vi "LDA_Analysis.vi"() -> (5 "Plug in titles":string[](array[string]), 7 "Plug in values":string[](array[string]))   [LabVIEW 2011]
uses:
  Controls/Save_Data.ctl
  Globals/LDA_meas_global_1.vi
  Globals/Plug_in_data_global.vi
  Globals/Meas_global.vi
  Globals/Constants_global.vi
  <vilib>/Analysis/NI_AALBase.lvlib
panel:
  in  "File Extension":string=".xls"
  out "Delta f":dbl
  in  "Refined Spectra":bool
  in  "No of estimates output":i32=300
  out "Autocorrelation":cluster{dbl, dbl, dbl[]}[](graph)
  in  "Mode":enum16{"Spectra", "Autocorrelation"}(ring)
  in  "Separation Character":string="\t"
  in  "Precision":i16=2
  out "Ch names":string[](array[string])
  out "Number or Good blocks":i32
  out "Resampled block length":i32
  out "Resampling Frequency":dbl
  in  "Output Directory":path
  in  "File":T1=enum."Save Data"
  out "Frequency Spectrum":cluster{dbl, dbl, dbl[]}[](graph)
  # "You must have just these two indicators on the connector pane of the vi"
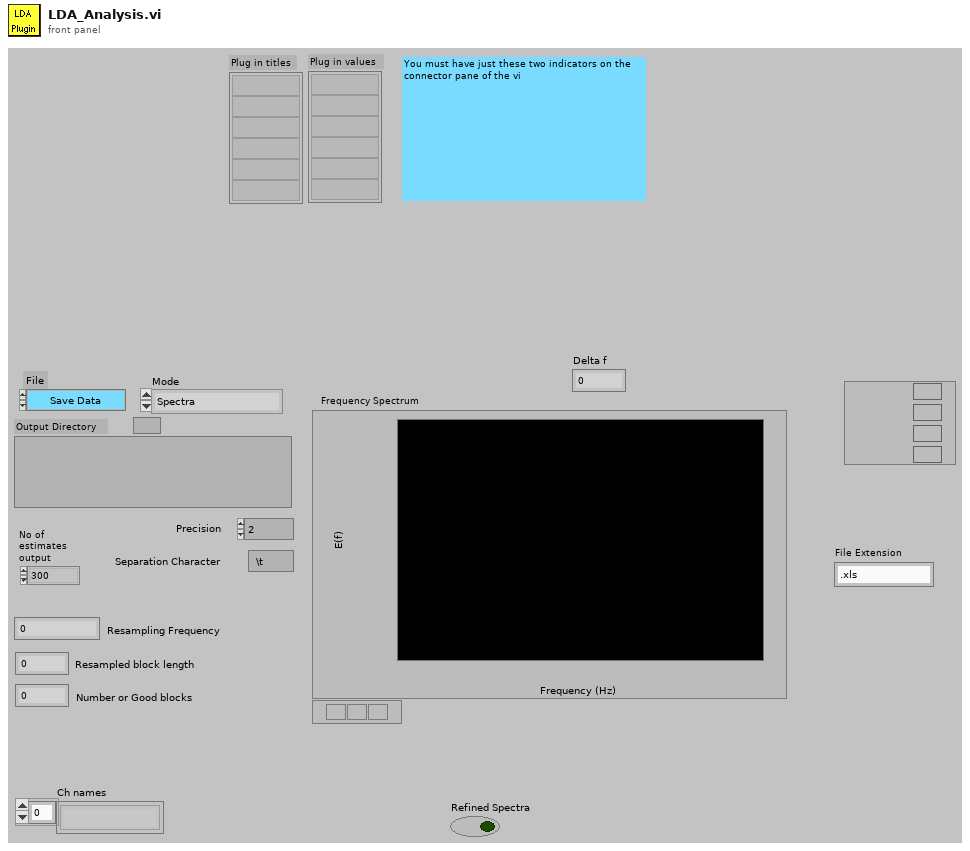
[diagram p1: front panel]
types:
  T1 = typedef "Save_Data.ctl" = enum16{"Save No Data", "Save Data"}
  T2 = enum32{"existing file", "new file", "new or existing file", "existing dir", "new dir", "new or existing dir", "existing file (use LLBs)", "new file (use LLBs)", "new or existing file (use LLBs)", "new or existing file or directory (use LLBs)"}
  T3 = typedef "Analysis_info_cluster.ctl" = cluster{"Colour":u32, "Inst type":T4, "Inst name":string, "Symbol":string, "Code name":string, "Extra Info":string, "Inst Array":T5, "Index":i32, "Voltage Index":i32, "Extra Titles":string[], "Extra Values":string[], "Eng Values":dbl[], "Time (ms)":dbl[], "TT / Voltage":dbl[], "U":dbl, "u^2":dbl, "u^3":dbl, "u^4":dbl, "Skew_u":dbl, "Kurt_u":dbl, "Mean % Err":dbl, "% u'/U":dbl}
  T4 = typedef "Inst_type.ctl" = enum16{"Propeller anemometer", "Raw voltage", "Pressure Transducer", "Pitot-static tube", "Preston tube", "Hot wire", "Cross wire 1", "Cross wire 2", "Generic Linear", "Generic Polynomial", "Generic BackPoly", "Fast FID", "Thermocouple", "Cold wire", "Pulsed Wire", "LDA Vel", "LDA Tran time", "LDA Arr time"}
  T5 = typedef "Instrument_Array.ctl" = enum16{"PWA", "LDA", "Analogue"}
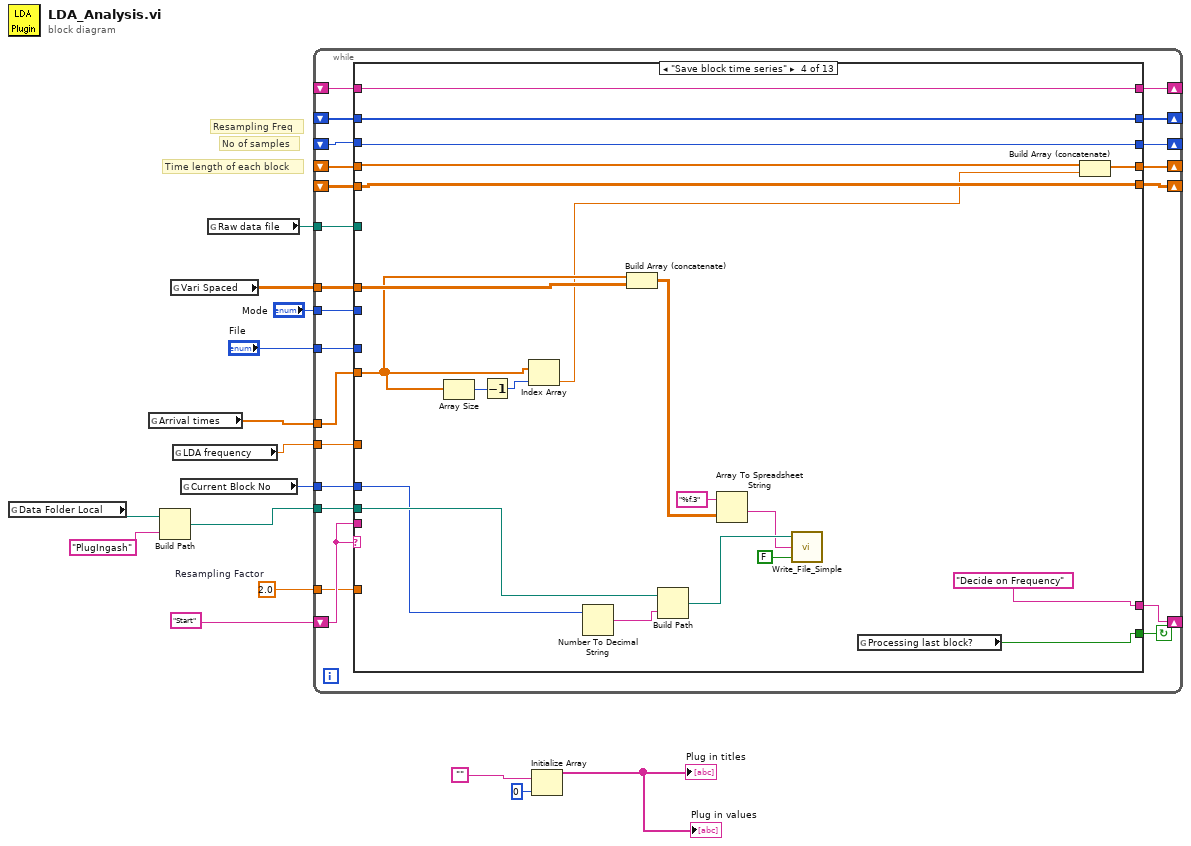
[diagram p0: block diagram]
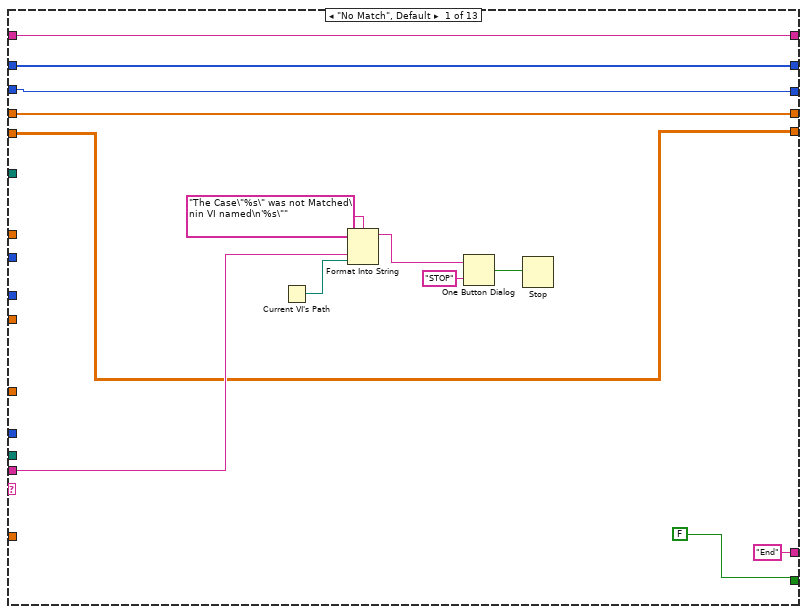
[diagram p2: hidden frame]
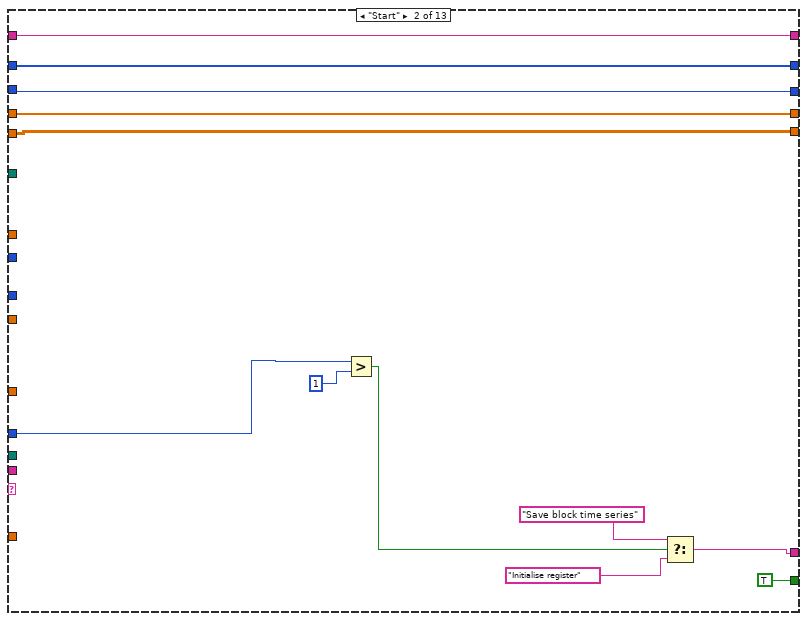
[diagram p3: hidden frame]
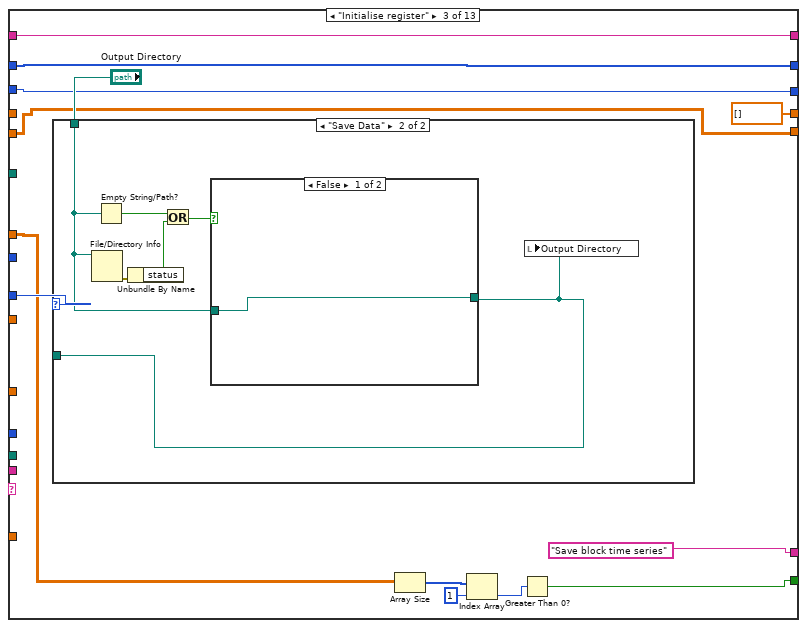
[diagram p4: hidden frame]
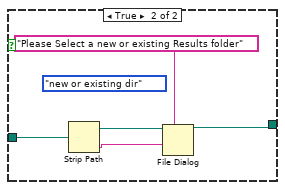
[diagram p6: hidden frame]
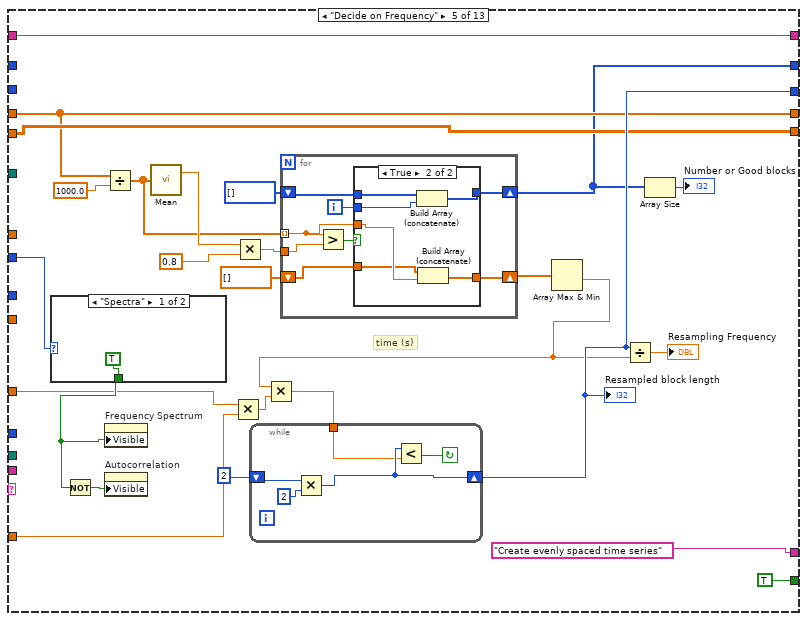
[diagram p7: hidden frame]
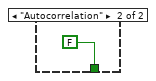
[diagram p8: hidden frame]
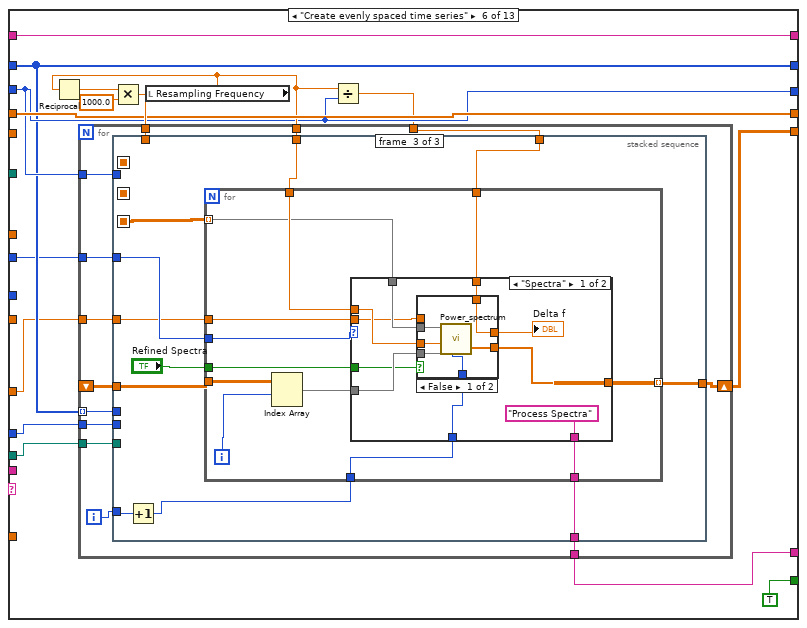
[diagram p10: hidden frame]
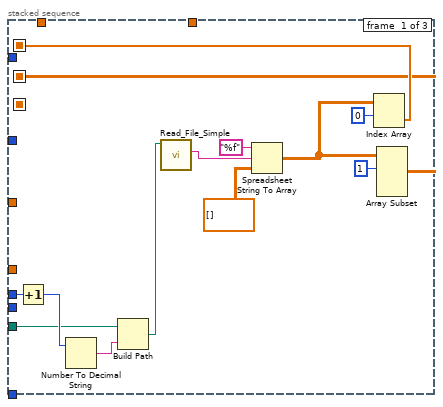
[diagram p11: hidden frame]
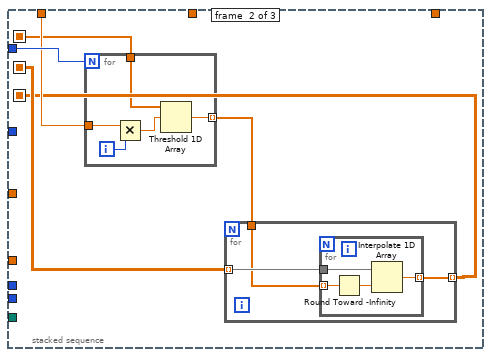
[diagram p12: hidden frame]
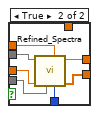
[diagram p13: hidden frame]
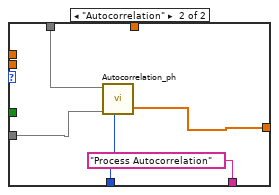
[diagram p14: hidden frame]
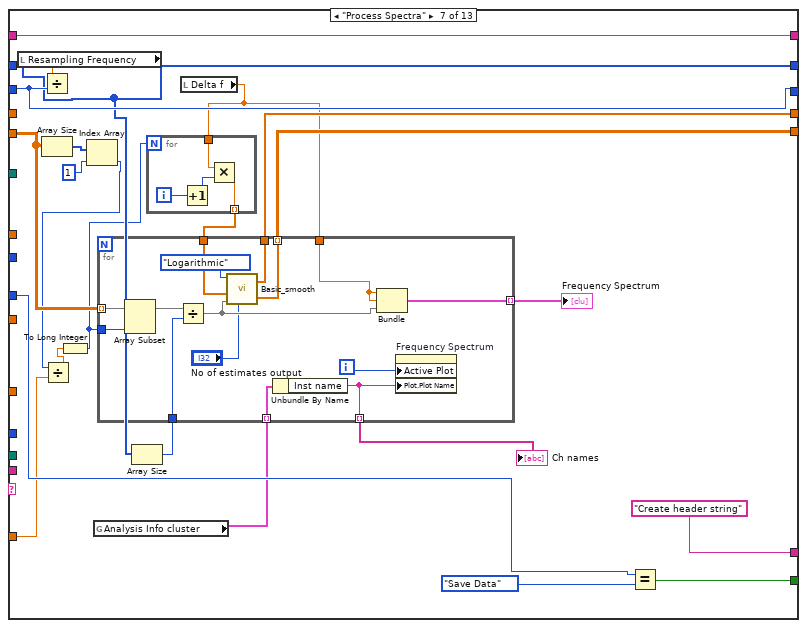
[diagram p15: hidden frame]
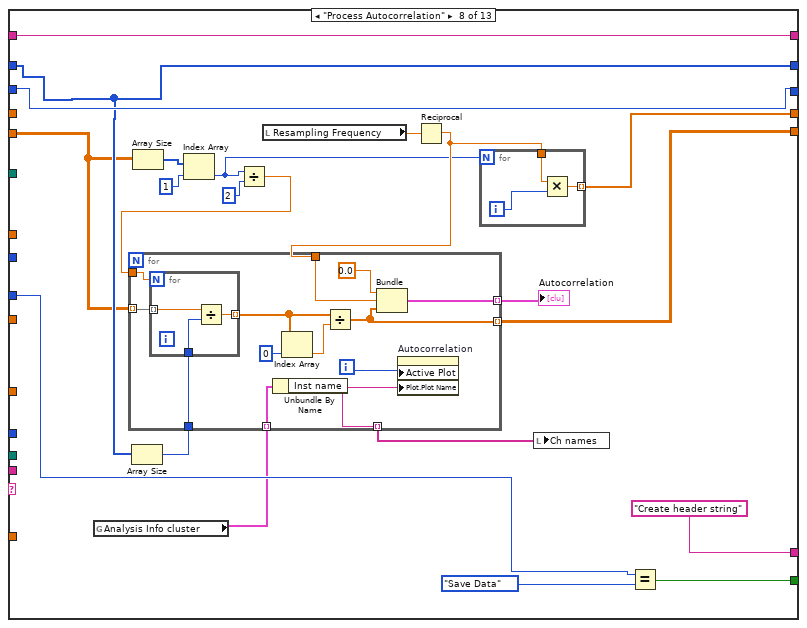
[diagram p16: hidden frame]
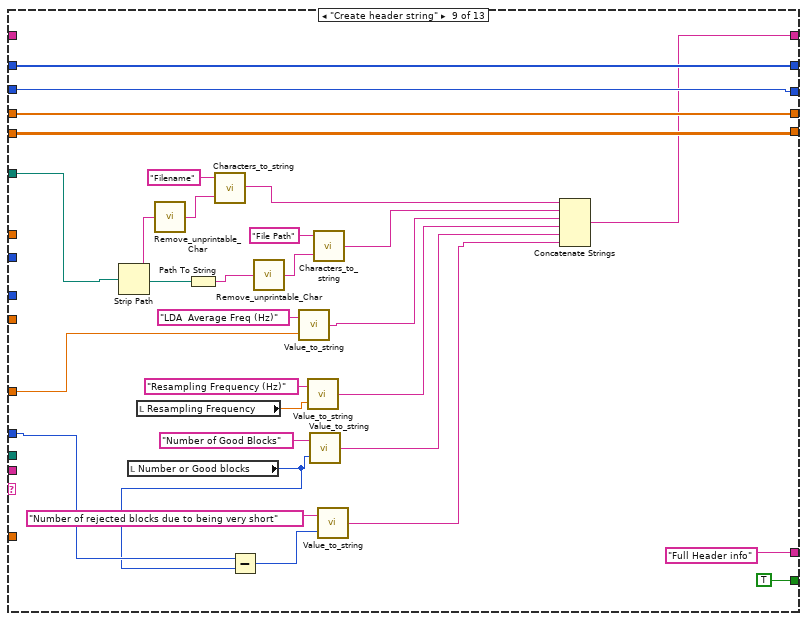
[diagram p17: hidden frame]
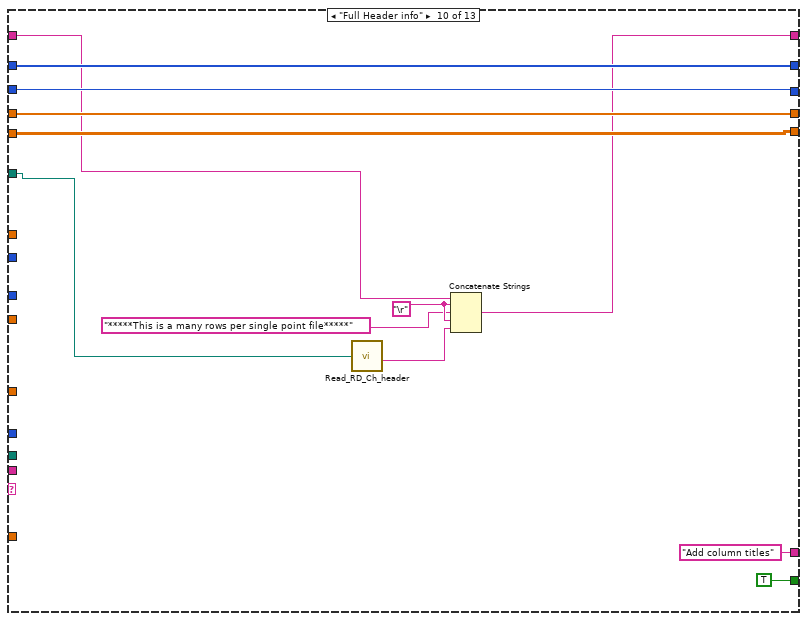
[diagram p18: hidden frame]
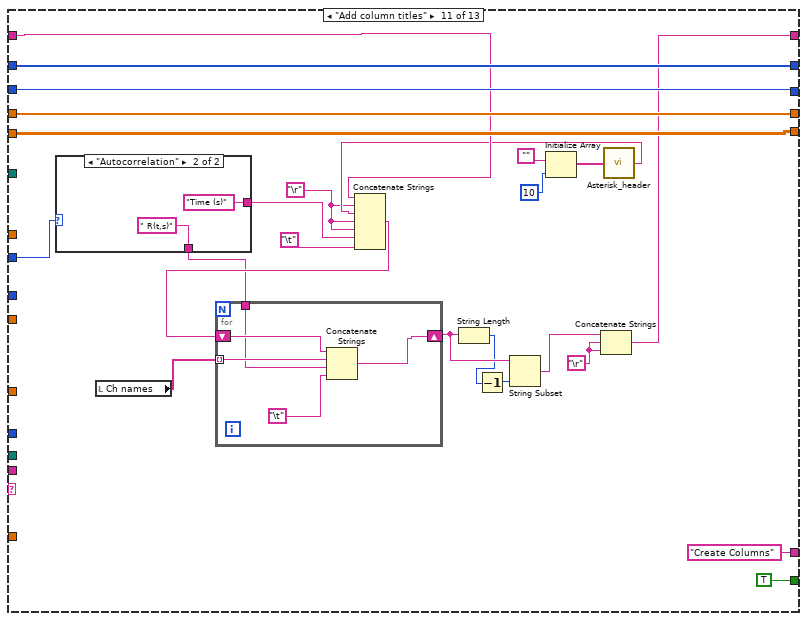
[diagram p19: hidden frame]
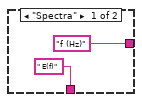
[diagram p20: hidden frame]
diagram:
  w1 = 2.0  # Resampling Factor
  # "No of samples"
  # "Time length of each block"
  # "Resampling Freq"
  n1 = global read "Constants_global.vi" "Data Folder Local"() -> (w7:path)
  n2 = global read "LDA_meas_global_1.vi" "Arrival times"() -> (w13:dbl[])
  n3 = Build Path(base path=w7, name or relative path="PlugIngash") -> (appended path=w6:path)
  n4 = global read "Plug_in_data_global.vi" "Vari Spaced"() -> (w14:dbl[][])
  n5 = global read "Meas_global.vi" "LDA frequency"() -> (w3:dbl)
  n6 = global read "Meas_global.vi" "Current Block No"() -> (w9:i32)
  n7 = global read "Meas_global.vi" "Raw data file"() -> (w4:path)
  n8 = while {
    shift-left: "Start" -> [w37]
    shift-right: [w34] -> _
    tunnel: w14 -> [w36]
    tunnel: w13 -> [w35]
    shift-right: [w32] -> _
    shift-left: _ -> [w31]
    shift-right: [w30] -> _
    shift-left: _ -> [w29]
    tunnel: w9 -> [w28]
    tunnel: w6 -> [w27]
    shift-right: [w26] -> _
    shift-left: _ -> [w25]
    tunnel: "File" -> [w24]
    shift-right: [w23] -> _
    shift-left: _ -> [w22]
    tunnel: w4 -> [w21]
    tunnel: w3 -> [w20]
    shift-right: [w19] -> _
    shift-left: _ -> [w18]
    tunnel: "Mode" -> [w17]
    tunnel: w1 -> [w16]
    stop <- w33 continue-if-true
    n9 = case shown="\"Save block time series\"" w37 {
      tunnel: ["End" ("t") w57 "Save block time series" ("t") "Decide on Frequency" ("t") "Create evenly spaced time series" ("t") w161 "Create header string" "Create header string" "Full Header info" ("t") "Add column titles" ("t") "Create Columns" ("t") "Save to file" ("t") "End" ("t")] -> w34
      tunnel: w37 -> [w46 _ _ _ _ _ _ _ _ _ _ _ _]
      tunnel: w36 -> [_ _ w67 w93 _ _ _ _ _ _ _ _ _]
      tunnel: w35 -> [_ _ _ w90 _ _ _ _ _ _ _ _ _]
      tunnel: [FALSE TRUE w63 w101 TRUE TRUE ("Processing last block?") w287 w328 TRUE ("Processing last block?") TRUE ("Processing last block?") TRUE ("Processing last block?") TRUE ("Processing last block?") FALSE] -> w33
      tunnel: [w43 w53 w70 w97 w128 w170 w283 w322 w355 w390 w414 w432 _] -> w32
      tunnel: w31 -> [w43 w53 w70 w97 w128 _ w276 w319 w355 w390 w414 w432 _]
      tunnel: [w41 w56 dbl[] [] w99 w124 w169 w279 w313 w356 w391 w415 w427 w488] -> w30
      tunnel: w29 -> [w41 w56 _ w100 w124 w169 _ _ w356 w391 w415 w427 w488]
      tunnel: w28 -> [_ w55 _ w106 _ w159 _ _ w364 _ _ _ _]
      tunnel: w27 -> [_ _ _ w107 _ w172 _ _ _ _ _ _ _]
      tunnel: [w42 w54 w71 w98 w129 w166 w290 w331 w357 w392 w416 w434 w489] -> w26
      tunnel: w25 -> [w42 w54 w71 w98 _ w166 w290 w331 w357 w392 w416 w434 w489]
      tunnel: w24 -> [_ _ w72 _ _ _ w288 w329 _ _ _ _ _]
      tunnel: [w40 w52 w69 w96 w118 w164 w282 w325 w358 w393 w417 w442 w487] -> w23
      tunnel: w22 -> [w40 w52 w69 w96 _ w164 w282 w325 w358 w393 w417 w442 w487]
      tunnel: w21 -> [_ _ _ _ _ _ _ _ w370 w383 _ _ w486]
      tunnel: w20 -> [_ _ _ _ w111 w160 _ _ w367 _ _ _ _]
      tunnel: [w39 w51 w68 w95 w116 w163 w286 w327 w354 w382 w410 w438 w479] -> w19
      tunnel: w18 -> [w39 w51 w68 w95 w116 w163 w286 w327 _ w389 w404 w439 w479]
      tunnel: w17 -> [_ _ _ _ w115 w162 _ _ _ _ w407 _ w476]
      tunnel: w16 -> [_ _ _ _ w110 _ w272 _ _ _ _ _ _]
      frame "No Match", Default {
        n10 = Current VI's Path() -> (path=w45:path)
        n11 = Format Into String(format string="The Case\"%s\" was not Matched\nin VI named\n'%s\"" ("Format String"), w46, w45) -> (resulting string=w49:string)  [unwired: 2 in, 1 out]
        n12 = One Button Dialog(message=w49, button name ("OK")="STOP") -> (true=w47:bool)
        n13 = Stop(stop? (T)=w47) -> ()
      }
      frame "Start" {
        n14 = Greater?(x=w55, y=1) -> (0:w59:bool)
        n15 = Select(t="Save block time series", s=w59, f="Initialise register") -> (s? t:f=w57:string)
      }
      frame "Initialise register" {
        n16 = case shown="\"Save Data\"" w72 {
          tunnel: [w76 w82] -> _
          tunnel: "Output Directory" -> [w76 w80]
          frame "Save No Data" {
          }
          frame "Save Data" {
            n17 = File/Directory Info(path=w80) -> (error out=w81:errorcluster)  [unwired: 1 in, 6 out]
            n18 = Empty String/Path?(string/path=w80) -> (empty?=w78:bool)
            n19 = Unbundle By Name(w81) -> ("status"=w79:bool)
            n20 = Or(x=w78, y=w79) -> (x .or. y?=w77:bool)
            n21 = case shown="False" w77 {
              tunnel: [w83 w88] -> w82
              tunnel: w80 -> [w83 w86]
              frame False {
              }
              frame True {
                (unwired) T2."new or existing dir" ("select mode (2)")
                n22 = Strip Path(path=w86) -> (stripped path=w85:path, name=w84:string)
                n23 = File Dialog(7:"Please Select a new or existing Results folder" ("prompt"), 9:w84, 11:w85) -> (3:w88:path)  [unwired: 1 in, 6 out]
              }
            }
            n24 = local write "Output Directory"(w82) -> ()
          }
        }
        n25 = Array Size(array=w67) -> (size(s)=w66:i32[])
        n26 = Index Array(array=w66, index=1) -> (element=w64:i32)
        n27 = Greater Than 0?(x=w64) -> (x > 0?=w63:bool)
      }
      frame "Save block time series" {
        n28 = Array Size(array=w90) -> (size(s)=w92:i32)
        n29 = Decrement(x=w92) -> (x-1=w91:i32)
        n30 = Index Array(array=w90, index=w91) -> (element=w89:dbl)
        n31 = Number To Decimal String(number=w106) -> (decimal integer string=w105:string)  [unwired: 1 out]
        n32 = Build Array (concatenate)(w90, w93) -> (w94:dbl[][])
        n33 = Build Path(base path=w107, name or relative path=w105) -> (appended path=w104:path)
        n34 = Array To Spreadsheet String(array=w94, 3:"%f.3" ("format string")) -> (spreadsheet string=w103:string)  [unwired: 1 out]
        n35 = call "Write_File_Simple.vi"("append to file? (new file:F)"=FALSE, "character string"=w103, "file path"=w104) -> ()  [unwired: 2 out]
        n36 = global read "Meas_global.vi" "Processing last block?"() -> (w101:bool)
        n37 = Build Array (concatenate)(w100, w89) -> (w99:dbl[])
      }
      frame "Decide on Frequency" {
        # "time (s)"
        n38 = case shown="\"Spectra\"" w115 {
          tunnel: [TRUE FALSE] -> w113
          frame "Spectra" {
          }
          frame "Autocorrelation" {
          }
        }
        n39 = Not(x=w113) -> (.not. x?=w114:bool)
        n40 = Divide(x=w124, y=1000.0) -> (x/y=w122:dbl[])
        n41 = property on="Frequency Spectrum" class="WFGraph (strict)"("Visible"=w113) -> ()  [unwired: 2 in, 2 out]
        n42 = property on="Autocorrelation" class="WFGraph (strict)"("Visible"=w114) -> ()  [unwired: 2 in, 2 out]
        n43 = call <vilib>:"Mean.vi"("X"=w122) -> ("mean"=w127:dbl)  [unwired: 1 out]
        n44 = Multiply(x=w111, y=w110) -> (x*y=w112:dbl)
        n45 = Multiply(x=w127, y=0.8) -> (x*y=w125:dbl)
        n46 = for {
          tunnel: w122 -> [w140] mode=indexing
          tunnel: w125 -> [w145]
          shift-right: [w141] -> w118
          shift-left: i32[] [] -> [w142]
          shift-right: [w138] -> w120
          shift-left: dbl[] [] -> [w139]
          i -> [w143]
          n47 = Greater?(x=w140, y=w145) -> (0:w144:bool)
          n48 = case shown="True" w144 {
            tunnel: w143 -> [_ w153]
            tunnel: w142 -> [w147 w152]
            tunnel: [w147 w151] -> w141
            tunnel: w140 -> [_ w150]
            tunnel: w139 -> [w146 w149]
            tunnel: [w146 w148] -> w138
            frame False {
            }
            frame True {
              n49 = Build Array (concatenate)(w152, w153) -> (w151:i32[])
              n50 = Build Array (concatenate)(w149, w150) -> (w148:dbl[])
            }
          }
        }
        n51 = Array Max & Min(array=w120) -> (min value=w119:dbl)  [unwired: 3 out]
        n52 = Multiply(x=w119, y=w112) -> (x*y=w131:dbl)
        n53 = while {
          shift-right: [w156] -> w129
          shift-left: 2 -> [w158]
          tunnel: w131 -> [w155]
          stop <- w154 continue-if-true
          n54 = Multiply(x=w158, y=2) -> (x*y=w156:i32)
          n55 = Less?(x=w156, y=w155) -> (x < y?=w154:bool)
        }
        "Resampled block length" <- w129
        n56 = Divide(x=w129, y=w119) -> (x/y=→"Resampling Frequency":dbl)
        n57 = Array Size(array=w118) -> (size(s)=→"Number or Good blocks":i32)
      }
      frame "Create evenly spaced time series" {
        n58 = local read "Resampling Frequency"() -> (w167:dbl)
        n59 = Reciprocal(x=w167) -> (1/x=w173:dbl)
        n60 = Multiply(x=w173, y=1000.0) -> (x*y=w171:dbl)
        n61 = Divide(x=w167, y=w166) -> (x/y=w165:dbl)
        n62 = for {
          tunnel: w172 -> [w187]
          tunnel: w166 -> [w186]
          tunnel: w171 -> [w185]
          shift-right: [w183] -> w170
          shift-left: _ -> [w184]
          tunnel: w167 -> [w182]
          tunnel: w165 -> [w181]
          tunnel: w164 -> [w179] mode=indexing
          tunnel: w162 -> [w178]
          tunnel: [w177] -> w161
          tunnel: w160 -> [w176]
          tunnel: w159 -> [w175]
          i -> [w180]
          n63 = stacked-sequence {
            seq-local: [w193 _ _] -> [_ w204 _]
            seq-local: [w190 _ _] -> [_ w202 _]
            seq-local: [_ w201 _] -> [_ _ w229]
            tunnel: w180 -> [_ _ w225]
            tunnel: w187 -> [w198 _ _]
            tunnel: w186 -> [_ w206 _]
            tunnel: w185 -> [_ w205 _]
            tunnel: w184 -> [_ _ w228]
            tunnel: [_ _ w227] -> w183
            tunnel: w182 -> [_ _ w226]
            tunnel: w181 -> [_ _ w219]
            tunnel: w179 -> [w188 _ _]
            tunnel: w178 -> [_ _ w223]
            tunnel: [_ _ w222] -> w177
            tunnel: w176 -> [_ _ w221]
            tunnel: w175 -> [_ _ _]
            frame #0 {
              n64 = Increment(x=w188) -> (x+1=w199:i32)
              n65 = Number To Decimal String(number=w199) -> (decimal integer string=w200:string)  [unwired: 1 out]
              n66 = Build Path(base path=w198, name or relative path=w200) -> (appended path=w197:path)
              n67 = call "Read_File_Simple.vi"("Filename"=w197) -> ("string"=w196:string)  [unwired: 2 in, 7 out]
              n68 = Spreadsheet String To Array(format string="%f", spreadsheet string=w196, array type (2D Dbl)=dbl[][] []) -> (array=w192:dbl[][])  [unwired: 1 out]
              n69 = Index Array(array=w192, index (row)=0) -> (element=w193:dbl[])  [unwired: 1 in]
              n70 = Array Subset(array=w192, index (row)=1 ("index")) -> (w190:dbl[][])  [unwired: 3 in]
            }
            frame #1 {
              n71 = for {
                N: w206 -> [_]
                tunnel: w205 -> [w217]
                tunnel: w204 -> [w216]
                tunnel: [w215] -> w203 mode=indexing
                i -> [w218]
                n72 = Multiply(x=w217, y=w218) -> (x*y=w214:dbl)
                n73 = Threshold 1D Array(2:w214, 3:w216) -> (0:w215:dbl)  [unwired: 1 out]
              }
              n74 = for {
                tunnel: [w209] -> w201 mode=indexing
                tunnel: w203 -> [w207]
                tunnel: w202 -> [w208] mode=indexing
                n75 = for {
                  tunnel: w208 -> [w213]
                  tunnel: w207 -> [w212] mode=indexing
                  tunnel: [w211] -> w209 mode=indexing
                  n76 = Round Toward -Infinity(1:w212) -> (0:w210:dbl)
                  n77 = Interpolate 1D Array(1:w210, 2:w213) -> (0:w211:dbl)
                }
              }
            }
            frame #2 {
              n78 = Increment(x=w225) -> (x+1=w224:i32)
              n79 = for {
                tunnel: w229 -> [w237] mode=indexing
                tunnel: [w236] -> w227 mode=indexing
                tunnel: w228 -> [w241]
                tunnel: w226 -> [w238]
                tunnel: w224 -> [w235]
                tunnel: w223 -> [w234]
                tunnel: [w233] -> w222
                tunnel: w221 -> [w232]
                tunnel: "Refined Spectra" -> [w231]
                tunnel: w219 -> [w230]
                i -> [w239]
                n80 = Index Array(array=w241, index (row)=w239) -> (element=w240:dbl[])  [unwired: 1 in]
                n81 = case shown="\"Spectra\"" w234 {
                  tunnel: w240 -> [w251 w268]
                  tunnel: w238 -> [w246 _]
                  tunnel: w237 -> [w247 w269]
                  tunnel: [w250 w267] -> w236
                  tunnel: w235 -> [w249 w266]
                  tunnel: ["Process Spectra" ("t") "Process Autocorrelation" ("t")] -> w233
                  tunnel: w232 -> [w245 _]
                  tunnel: w231 -> [w244 _]
                  tunnel: w230 -> [w242 _]
                  frame "Spectra" {
                    n82 = case shown="False" w244 {
                      tunnel: w251 -> [w257 w261]
                      tunnel: [w256 w263] -> w250
                      tunnel: w249 -> [w255 w260]
                      tunnel: w247 -> [w254 w264]
                      tunnel: w246 -> [w253 w262]
                      tunnel: w245 -> [_ w259]
                      tunnel: [w252 w258] -> w243
                      tunnel: w242 -> [w252 _]
                      frame False {
                        n83 = call "Power_spectrum.vi"("U"=w254, "Sampling frequency"=w253, "Spectrum input array"=w257, "Block No"=w255) -> ("Spectrum output array"=w256:dbl[])  [unwired: 1 in, 1 out]
                      }
                      frame True {
                        n84 = call "Refined_Spectra.vi"("Block No"=w260, "LDA Frequency"=w259, "Spectrum input array"=w261, "Sampling frequency"=w262, "X"=w264) -> ("Spectrum"=w263:dbl[], "Delta f"=w258:dbl)  [unwired: 5 in]
                      }
                    }
                    "Delta f" <- w243
                  }
                  frame "Autocorrelation" {
                    n85 = call "Autocorrelation_ph.vi"("X"=w269, "Autocorrelation of X"=w268, "Block No"=w266) -> ("Autocorrelation of X"=w267:dbl[])  [unwired: 2 in, 1 out]
                  }
                }
              }
            }
          }
        }
      }
      frame "Process Spectra" {
        (unwired) FALSE
        n86 = local read "Resampling Frequency"() -> (w291:dbl)
        n87 = Divide(x=w291, y=w290) -> ()  [unwired: 1 out]
        n88 = Array Size(array=w276) -> (size(s)=w278:i32[])
        n89 = Index Array(array=w278, index=1) -> (element=w273:i32)
        n90 = Divide(x=w273, y=w272) -> (x/y=w271:dbl)
        n91 = To Long Integer(number=w271) -> (32bit integer=w270:i32)
        n92 = global read "Meas_global.vi" "Analysis Info cluster"() -> (w284:T3[])
        n93 = Array Size(array=w282) -> (size(s)=w281:i32)
        n94 = local read "Delta f"() -> (w275:dbl)
        n95 = for {
          N: w270 -> [_]
          tunnel: w275 -> [w294]
          tunnel: [w293] -> w280 mode=indexing
          i -> [w296]
          n96 = Increment(x=w296) -> (x+1=w295:i32)
          n97 = Multiply(x=w294, y=w295) -> (x*y=w293:dbl)
        }
        n98 = for {
          tunnel: w276 -> [w298] mode=indexing
          tunnel: w281 -> [w311]
          tunnel: [w310] -> w274 mode=indexing
          tunnel: w284 -> [w308] mode=indexing
          tunnel: [w307] -> w285 mode=indexing
          tunnel: [w302] -> w283 mode=indexing
          tunnel: w280 -> [w305]
          tunnel: [w301] -> w279
          tunnel: w275 -> [w300]
          tunnel: w270 -> [w297]
          i -> [w309]
          n99 = Array Subset(array=w298, length=w297) -> (w299:dbl[])  [unwired: 1 in]
          n100 = Divide(x=w299, y=w311) -> (x/y=w306:dbl[])
          n101 = call "Basic_smooth.vi"("Smoothing"=enum16{"Linear", "Logarithmic"}."Logarithmic", "X array in"=w305, "Y array in"=w306, "No of estimates output"="No of estimates output") -> ("X array Out"=w301:dbl[], "Y array Out"=w302:dbl[])  [unwired: 1 out]
          n102 = Unbundle By Name(w308) -> ("Inst name"=w307:string)
          n103 = Bundle("Delta f"=w300, "Delta f"=w300, w306) -> (w310:cluster{"Delta f":dbl, "Delta f":dbl, dbl[]})  [unwired: 1 out]
          n104 = property on="Frequency Spectrum" class="WFGraph (strict)"("Active Plot"=w309, "Plot.Plot Name"=w307) -> ()  [unwired: 2 in, 2 out]
        }
        "Frequency Spectrum" <- w274
        "Ch names" <- w285
        n105 = Equal?(x=w288, y=Save_Data."Save Data" ("File")) -> (x = y?=w287:bool)
      }
      frame "Process Autocorrelation" {
        (unwired) FALSE
        n106 = global read "Meas_global.vi" "Analysis Info cluster"() -> (w326:T3[])
        n107 = Array Size(array=w325) -> (size(s)=w324:i32)
        n108 = Array Size(array=w319) -> (size(s)=w318:i32[])
        n109 = Index Array(array=w318, index=1) -> (element=w312:i32)
        n110 = Divide(x=w312, y=2) -> (x/y=w315:dbl)
        n111 = local read "Resampling Frequency"() -> (w323:dbl)
        n112 = Reciprocal(x=w323) -> (1/x=w314:dbl)
        n113 = for {
          tunnel: w314 -> [w348]
          tunnel: w319 -> [w347] mode=indexing
          tunnel: w324 -> [w346]
          tunnel: [w345] -> w320 mode=indexing
          tunnel: w326 -> [w344] mode=indexing
          tunnel: [w339] -> w322 mode=indexing
          tunnel: [w337] -> w321 mode=indexing
          tunnel: w315 -> [w336]
          i -> [w338]
          n114 = for {
            N: w336 -> [_]
            tunnel: w347 -> [w351] mode=indexing
            tunnel: w346 -> [w350]
            tunnel: [w349] -> w341 mode=indexing
            n115 = Divide(x=w351, y=w350) -> (x/y=w349:dbl)
          }
          n116 = Unbundle By Name(w344) -> ("Inst name"=w337:string)
          n117 = Index Array(array=w341, index=0) -> (element=w340:dbl)
          n118 = Divide(x=w341, y=w340) -> (x/y=w339:dbl[])
          n119 = Bundle(0.0, w348, w339) -> (w345:cluster{dbl, dbl, dbl[]})  [unwired: 1 out]
          n120 = property on="Autocorrelation" class="WFGraph (strict)"("Active Plot"=w338, "Plot.Plot Name"=w337) -> ()  [unwired: 2 in, 2 out]
        }
        "Autocorrelation" <- w320
        n121 = for {
          N: w312 -> [_]
          tunnel: w314 -> [w335]
          tunnel: [w333] -> w313 mode=indexing
          i -> [w334]
          n122 = Multiply(x=w335, y=w334) -> (x*y=w333:dbl)
        }
        n123 = local write "Ch names"(w321) -> ()
        n124 = Equal?(x=w329, y=Save_Data."Save Data" ("File")) -> (x = y?=w328:bool)
      }
      frame "Create header string" {
        n125 = Strip Path(path=w370) -> (stripped path=w374:path, name=w378:string)
        n126 = local read "Number or Good blocks"() -> (w363:i32)
        n127 = local read "Resampling Frequency"() -> (w366:dbl)
        n128 = call "Remove_unprintable_Char.vi"("Input String"=w378) -> ("Output String"=w377:string)
        n129 = Path To String(path=w374) -> (string=w373:string)
        n130 = call "Characters_to_string.vi"("Characters to write"=w377, "Label for characters"="Filename") -> ("Output string"=w372:string)
        n131 = Subtract(x=w364, y=w363) -> (x-y=w362:i32)
        n132 = call "Remove_unprintable_Char.vi"("Input String"=w373) -> ("Output String"=w376:string)
        n133 = call "Value_to_string.vi"("Value"=w367, "Label for value"="LDA  Average Freq (Hz)") -> ("Output string"=w381:string)  [unwired: 1 in]
        n134 = call "Value_to_string.vi"("Value"=w366, "Label for value"="Resampling Frequency (Hz)") -> ("Output string"=w361:string)  [unwired: 1 in]
        n135 = call "Value_to_string.vi"("Value"=w363, "Label for value"="Number of Good Blocks") -> ("Output string"=w360:string)  [unwired: 1 in]
        n136 = call "Characters_to_string.vi"("Characters to write"=w376, "Label for characters"="File Path") -> ("Output string"=w371:string)
        n137 = call "Value_to_string.vi"("Value"=w362, "Label for value"="Number of rejected blocks due to being very short") -> ("Output string"=w359:string)  [unwired: 1 in]
        n138 = Concatenate Strings(w372, w371, w381, w361, w360, w359) -> (w354:string)
      }
      frame "Full Header info" {
        w386 = "\r"
        n139 = call "Read_RD_Ch_header.vi"("Raw data file"=w383) -> ("Ch string"=w384:string)  [unwired: 3 out]
        n140 = Concatenate Strings(w389, w386, "*****This is a many rows per single point file*****", w386, w384) -> (w382:string)
      }
      frame "Add column titles" {
        w398 = "\r"
        w399 = "\r"
        n141 = case shown="\"Autocorrelation\"" w407 {
          tunnel: ["f (Hz)" "Time (s)"] -> w406
          tunnel: [" E(f)" " R(t,s)"] -> w405
          frame "Spectra" {
          }
          frame "Autocorrelation" {
          }
        }
        n142 = local read "Ch names"() -> (w412:string[])
        n143 = Initialize Array("", 10) -> (w403:string[])
        n144 = call "Asterisk_header.vi"("Channel names"=w403) -> ("Header string"=w400:string)
        n145 = Concatenate Strings(w404, w398, w400, w398, w398, w406, "\t") -> (w411:string)
        n146 = for {
          shift-right: [w423] -> w397
          shift-left: w411 -> [w425]
          tunnel: w412 -> [w426] mode=indexing
          tunnel: w405 -> [w422]
          n147 = Concatenate Strings(w425, w426, w422, "\t") -> (w423:string)
        }
        n148 = String Length(string=w397) -> (length=w394:i32)
        n149 = Decrement(x=w394) -> (x-1=w395:i32)
        n150 = String Subset(string=w397, length (rest)=w395) -> (substring=w396:string)  [unwired: 1 out]
        n151 = Concatenate Strings(w396, w399, w399) -> (w410:string)
      }
      frame "Create Columns" {
        n152 = Array Size(array=w432) -> (size(s)=w430:i32[])
        n153 = Index Array(array=w430, index=0) -> (element=w429:i32)
        n154 = Decrement(x=w429) -> (x-1=w428:i32)
        n155 = for {
          shift-right: [w456] -> w437
          shift-left: "" -> [w451]
          tunnel: "Separation Character" -> [w444]
          tunnel: w432 -> [w454]
          tunnel: w428 -> [w450]
          tunnel: "Precision" -> [w448]
          tunnel: "Precision" -> [w447]
          tunnel: w427 -> [w443] mode=indexing
          i -> [w449]
          n156 = Index Array(array=w454, index (col)=w449) -> (element=w453:dbl[])  [unwired: 1 in]
          n157 = Number To Fractional String(number=w443, precision (6)=w447) -> (F-format string=w446:string)  [unwired: 2 out]
          n158 = Concatenate Strings(w446, w444) -> (w445:string)
          n159 = for {
            shift-right: [w463] -> w452
            shift-left: w445 -> [w465]
            tunnel: w444 -> [w462]
            tunnel: w453 -> [w457] mode=indexing
            tunnel: w450 -> [w460]
            tunnel: w448 -> [w458]
            i -> [w461]
            n160 = Equal?(x=w461, y=w460) -> (x = y?=w459:bool)
            n161 = Number To Exponential String(number=w457, precision (6)=w458) -> (E-format string=w464:string)  [unwired: 2 out]
            n162 = case shown="True" w459 {
              tunnel: w465 -> [w469 w472]
              tunnel: w464 -> [w468 w471]
              tunnel: [w467 w470] -> w463
              tunnel: w462 -> [w466 _]
              frame False {
                n163 = Concatenate Strings(w469, w468, w466) -> (w467:string)
              }
              frame True {
                n164 = Concatenate Strings(w472, w471) -> (w470:string)
              }
            }
          }
          n165 = Concatenate Strings(w451, w452, "\r") -> (w456:string)
        }
        n166 = Concatenate Strings(w439, w437) -> (w438:string)
      }
      frame "Save to file" {
        w481 = TRUE  # advisory dialog? (display:T)
        n167 = case shown="\"Spectra\"" w476 {
          tunnel: ["Spec_" ("string") "Auto_" ("string")] -> w477
          frame "Spectra" {
          }
          frame "Autocorrelation" {
          }
        }
        n168 = Strip Path(path=w486) -> (name=w484:string)  [unwired: 1 out]
        n169 = local read "Output Directory"() -> (w485:path)
        n170 = Concatenate Strings(w477, w484) -> (w475:string)
        n171 = call "Add_filename_suffix.vi"("Filename"=w475, "Suffix to add"="File Extension") -> ("Filename out"=w473:string)  [unwired: 3 out]
        n172 = Build Path(base path=w485, name or relative path=w473) -> (appended path=w483:path)
        n173 = call "Create_directory_path.vi"("Path name"=w483) -> ("Path name Out"=w482:path)  [unwired: 1 in, 1 out]
        n174 = call "Write_Characters_To_File.vi"("file path (dialog if empty)"=w482, "advisory dialog? (display:T)"=w481, "character string"=w479, "append to file? (new file:F)"=FALSE) -> ()  [unwired: 1 in, 4 out]
      }
    }
  }
  n175 = Initialize Array("", 0) -> (→"Plug in values" →"Plug in titles":string[])
